vi "FrequenzgeneratorInit.vi"(8 "Error_in":errorcluster, 11 "VISA Name FG in(FG)":refnum<visa-resource-name>="USB0::0x0957::0x0407::MY44043889::INSTR") -> (0 "Error_out":errorcluster)   [LabVIEW 2016]
doc: "Mit diesem VI wird der Frequenzgenerator Agilent 33220A initialisiert."
uses:
  <instrlib>/agilent_33xxx_series/Agilent 33XXX Series/Agilent 33XXX Series.lvlib
panel:
  in  "Amplitude (0,05)":dbl=0.05
  in  "Frequency (50 Hz)":dbl=50.0
  in  "Waveform Function (1: Sine)":u16(ring)=1 items=["DC", "Sine", "Square", "Triangle", "Ramp", "Pulse", "Noise", "Sinc", "Negative Ramp", "Exponential Rise", "Exponential Fall", "Cardiac"]
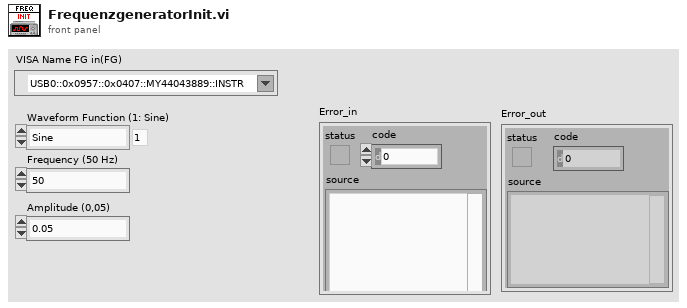
[diagram p1: front panel]
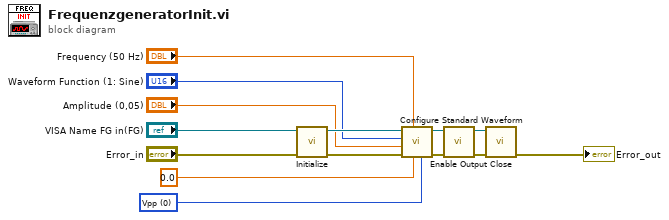
[diagram p0: block diagram]
diagram:
  w5 = u16 0 items=["Vpp", "Vrms", "dB"] ("Unit (0: Vpp)")
  n1 = call <instrlib>:"Initialize.vi"("error in (no error)"="Error_in", "VISA resource name"="VISA Name FG in(FG)") -> ("error out"=w11:errorcluster, "VISA resource name out"=w10:refnum<visa-resource-name>)  [unwired: 8 in]
  n2 = call <instrlib>:"Configure Standard Waveform.vi"("Unit (0: Vpp)"=w5, "DC Offset (0.00 V)"=0.0, "Frequency (1000 Hz)"="Frequency (50 Hz)", "error in (no error)"=w11, "Amplitude (1)"="Amplitude (0,05)", "Waveform Function (1: Sine)"="Waveform Function (1: Sine)", "VISA resource name"=w10) -> ("error out"=w9:errorcluster, "VISA resource name out"=w4:refnum<visa-resource-name>)  [unwired: 3 in]
  n3 = call <instrlib>:"Enable Output.vi"("error in (no error)"=w9, "VISA resource name"=w4) -> ("error out"=w14:errorcluster, "VISA resource name out"=w1:refnum<visa-resource-name>)  [unwired: 8 in]
  n4 = call <instrlib>:"Close.vi"("error in (no error)"=w14, "VISA resource name"=w1) -> ("error out"=→"Error_out":errorcluster)  [unwired: 9 in]
